vi "LBCB_Conversions.vi"(4 "Transformation Matrix":dbl[][](array[numeric]), 5 "Type":u16, 6 "Motion Center":dbl[](array[numeric]), 7 "Size":u16, 8 "error in (no error)":errorcluster, 9 "Error Log \nFilename":string, 10 "Conversion Type":T1, 11 "Input":dbl[](array[numeric])) -> (0 "error out":errorcluster, 1 "Output":dbl[](array[numeric]))   [LabVIEW 2013]
uses:
  LBCB_Conversions_Actions.ctl
  <vilib>/Analysis/baseanly.llb/A x Vector.vi
  <vilib>/Analysis/baseanly.llb/Real Inverse Matrix.vi
  DLL/LBCB_Conversions.dll
  <vilib>/Analysis/NI_AALBase.lvlib
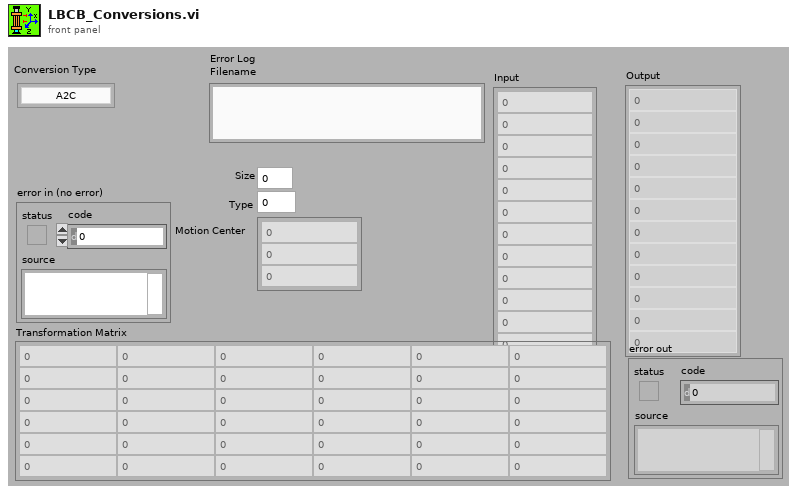
[diagram p1: front panel]
types:
  T1 = typedef "LBCB_Conversions_Actions.ctl" = enum16{"A2C", "C2A", "Set Log Filename", "Init"}
  T2 = typedef "NI_Matrix.lvlib/RealMatrix.ctl" = dbl[][]
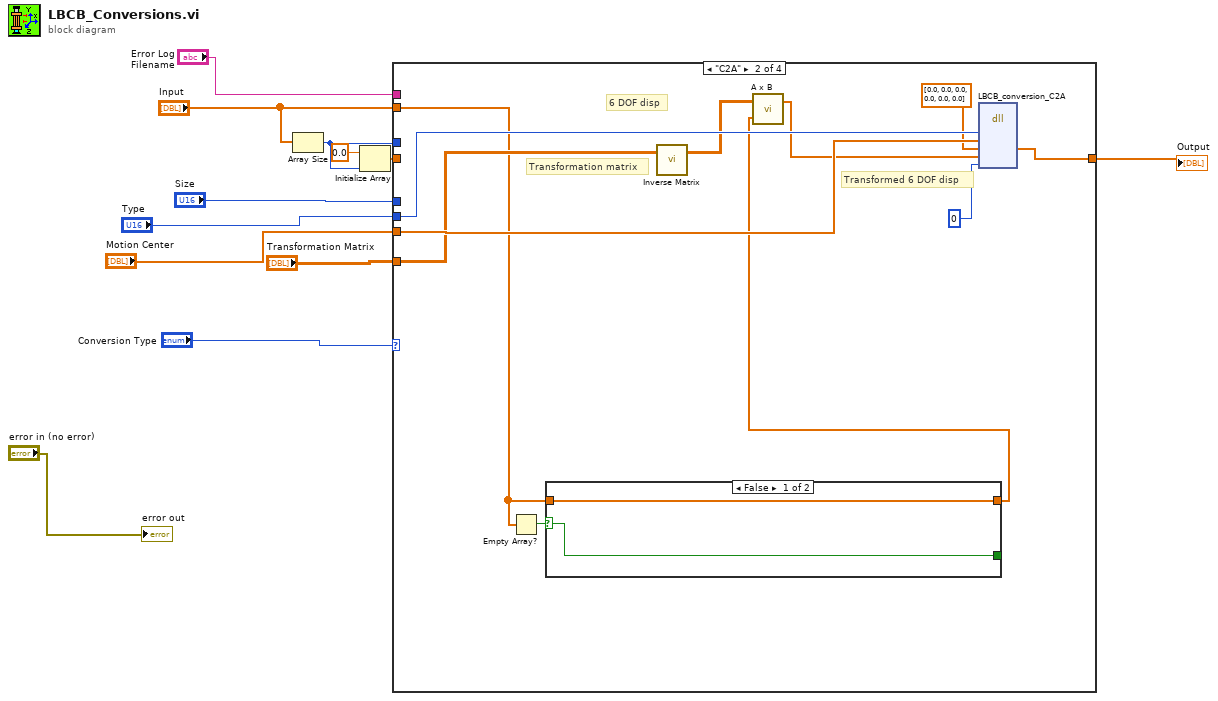
[diagram p0: block diagram]
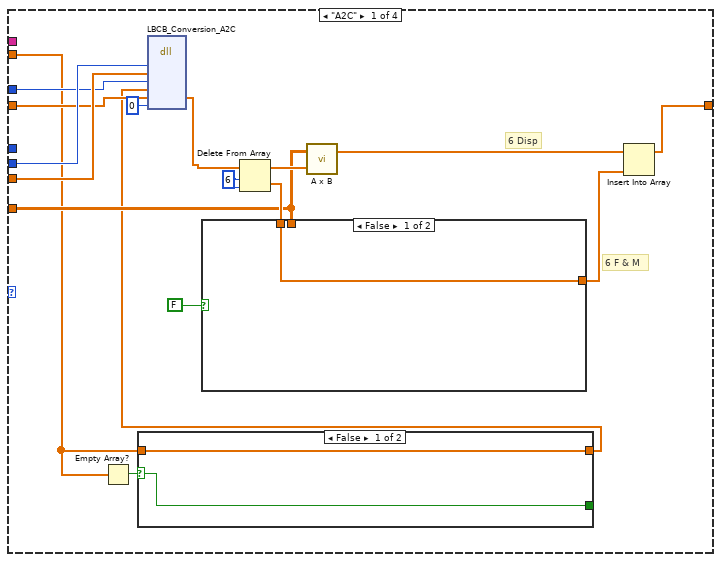
[diagram p2: hidden frame]
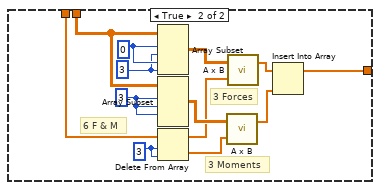
[diagram p3: hidden frame]
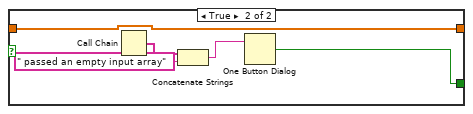
[diagram p4: hidden frame]
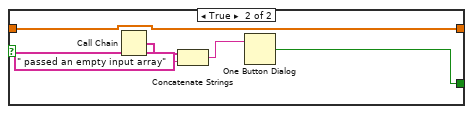
[diagram p5: hidden frame]
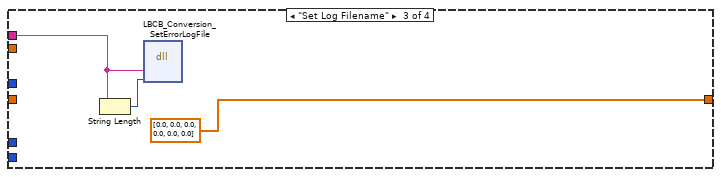
[diagram p6: hidden frame]
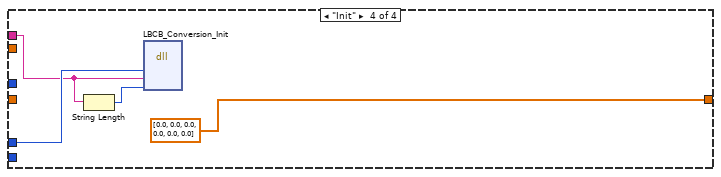
[diagram p7: hidden frame]
diagram:
  n1 = Array Size(array="Input") -> (size(s)=w9:i32)
  n2 = Initialize Array(0.0, w9) -> (w10:dbl[])
  n3 = case shown="\"C2A\"" "Conversion Type" {
    tunnel: "Input" -> [w15 w51 _ _]
    tunnel: [w17 w61 dbl[] [0.0, 0.0, 0.0, 0.0, 0.0, 0.0] dbl[] [0.0, 0.0, 0.0, 0.0, 0.0, 0.0]] -> w8
    tunnel: "Size" -> [_ _ _ w74]
    tunnel: "Type" -> [w29 w60 _ _]
    tunnel: "Motion Center" -> [w28 w59 _ _]
    tunnel: w10 -> [w27 _ _ _]
    tunnel: w9 -> [w26 _ _ _]
    tunnel: "Transformation Matrix" -> [w18 w55 _ _]
    tunnel: "Error Log \nFilename" -> [_ _ w69 w73]
    frame "A2C" {
      w20 = 6
      # "6 F & M"
      # "6 Disp"
      n4 = Empty Array?(array=w15) -> (empty?=w16:bool)
      n5 = case shown="False" w16 {
        selector: w16 -> [w45 _]
        tunnel: [w45 w47] -> _
        tunnel: w15 -> [w44 w46]
        tunnel: [w44 w46] -> w14
        frame False {
        }
        frame True {
          n6 = Call Chain() -> (call chain=w50:string[])
          n7 = Concatenate Strings(w50, " passed an empty input array" ("string")) -> (w49:string)
          n8 = One Button Dialog(message=w49) -> (true=w47:bool)  [unwired: 1 out]
        }
      }
      n9 = dll-call lib="C:/Users/mbletzin/Desktop/Work/NewLbcbConversionDll/DLL/LBCB_Conversions.dll" fn="LBCB_Conversion_A2C"("type"=w29, "motion_center"=w28, "length"=w26, "sensor_reading"=w14, "cartesian_value"=w27, "error"=0) -> ("cartesian_value"=w19:dbl[])  [unwired: 6 in, 5 out]
      n10 = Delete From Array(array=w19, length=w20, index=w20) -> (deleted portion=w23:dbl[], array with subset deleted=w21:dbl[])
      n11 = case shown="False" FALSE {
        tunnel: [w30 w43] -> w24
        tunnel: w23 -> [w30 w32]
        tunnel: w18 -> [_ w31]
        frame False {
        }
        frame True {
          w34 = 3
          w35 = 3
          w36 = 0
          w33 = 3
          # "3 Forces"
          # "3 Moments"
          # "6 F & M"
          n12 = Array Subset(array=w31, index (row)=w36, length (row)=w35, index (col)=w36, length (col)=w35) -> (w37:dbl[][])
          n13 = Array Subset(array=w31, index (row)=w34, length (row)=w34, index (col)=w34) -> (w39:dbl[][])  [unwired: 1 in]
          n14 = Delete From Array(array=w32, length=w33, index=w33) -> (deleted portion=w40:dbl[], array with subset deleted=w38:dbl[])
          n15 = call-poly <vilib>:"A x B.vi"("Vector"=w40, "A"=w39) -> ("A x Vector"=w42:dbl[])  [unwired: 1 out]
          n16 = call-poly <vilib>:"A x B.vi"("Vector"=w38, "A"=w37) -> ("A x Vector"=w41:dbl[])  [unwired: 1 out]
          n17 = Insert Into Array(array=w41, new element=w42) -> (w43:dbl[])  [unwired: 1 in]
        }
      }
      n18 = call-poly <vilib>:"A x B.vi"("Vector"=w21, "A"=w18) -> ("A x Vector"=w22:dbl[])  [unwired: 1 out]
      n19 = Insert Into Array(array=w22, new element=w24) -> (w17:dbl[])  [unwired: 1 in]
    }
    frame "C2A" {
      # "Transformation matrix"
      # "Transformed 6 DOF disp"
      # "6 DOF disp"
      n20 = Empty Array?(array=w51) -> (empty?=w53:bool)
      n21 = case shown="False" w53 {
        selector: w53 -> [w63 _]
        tunnel: [w63 w65] -> _
        tunnel: w51 -> [w62 w64]
        tunnel: [w62 w64] -> w52
        frame False {
        }
        frame True {
          n22 = Call Chain() -> (call chain=w68:string[])
          n23 = Concatenate Strings(w68, " passed an empty input array" ("string")) -> (w67:string)
          n24 = One Button Dialog(message=w67) -> (true=w65:bool)  [unwired: 1 out]
        }
      }
      n25 = call-poly <vilib>:"Inverse Matrix.vi"("Input Matrix"=w55) -> ("Inverse Matrix"=w56:T2)  [unwired: 1 in, 1 out]
      n26 = call-poly <vilib>:"A x B.vi"("Vector"=w52, "A"=w56) -> ("A x Vector"=w54:dbl[])  [unwired: 1 out]
      n27 = dll-call lib="C:/Users/mbletzin/Desktop/Work/NewLbcbConversionDll/DLL/LBCB_Conversions.dll" fn="LBCB_conversion_C2A"("type"=w60, "motion_center"=w59, "sensor_reading"=dbl[] [0.0, 0.0, 0.0, 0.0, 0.0, 0.0], "cartesian_value"=w54, "error"=0) -> ("sensor_reading"=w61:dbl[])  [unwired: 5 in, 5 out]
    }
    frame "Set Log Filename" {
      n28 = String Length(string=w69) -> (length=w70:i32)
      n29 = dll-call lib="C:/Users/mbletzin/Desktop/Work/NewLbcbConversionDll/DLL/LBCB_Conversions.dll" fn="LBCB_Conversion_SetErrorLogFile"("filename"=w69, "length"=w70) -> ()  [unwired: 5 in, 3 out]
    }
    frame "Init" {
      n30 = String Length(string=w73) -> (length=w72:i32)
      n31 = dll-call lib="C:/Users/mbletzin/Desktop/Work/NewLbcbConversionDll/DLL/LBCB_Conversions.dll" fn="LBCB_Conversion_Init"("size"=w74, "filename"=w73, "length"=w72) -> ()  [unwired: 5 in, 4 out]
    }
  }
  "Output" <- w8
  "error out" <- "error in (no error)"
